vi "configure.vi"(7 "httpRequestID":u32) -> ()   [LabVIEW 2011]
doc: "This VI is a state machine that can be ran from a Browser."
uses:
  server/database/Users/User Record.ctl
  <vilib>/wsapi/NI_WebServices.lvlib
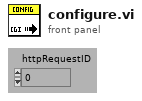
[diagram p1: front panel]
types:
  T1 = typedef "User Record.ctl" = cluster{"ixUser":i32, "sxUsername":string, "sLastName":string, "sFirstName":string, "sEmail":string, "sPassword":string, "tLoginTime":timestamp, "sLoginComputer":string, "fAdministrator":bool, "fRunSequences":bool, "fModifySequences":bool, "fRunScenarios":bool, "fModifyScenarios":bool, "fModifyTemplates":bool, "fModifyUsers":bool, "fModifyStations":bool, "fModifyFields":bool}
  T2 = typedef "Connection Refnum.ctl" = cluster{"Environment Handle":i32, "Connection Handle":i32}
  T3 = typedef "Keyed Array.ctl" = cluster{"keys":string[], "values":string[]}
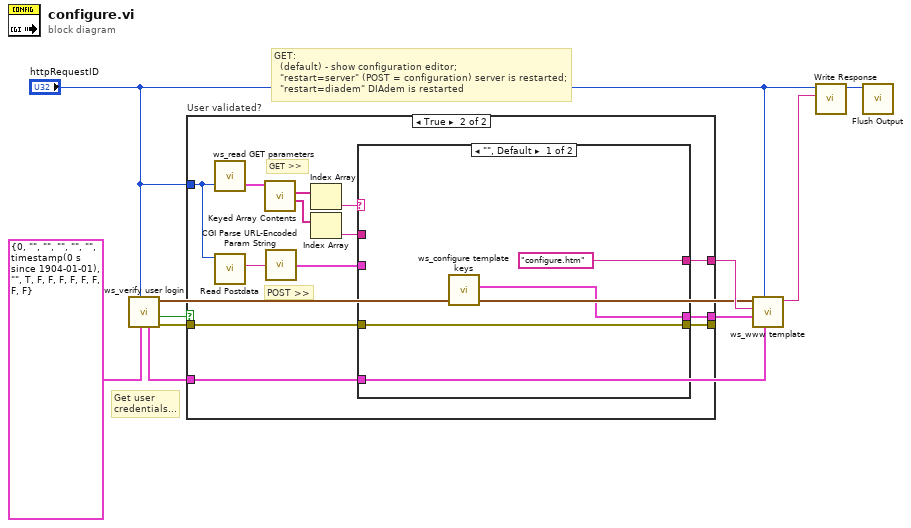
[diagram p0: block diagram]
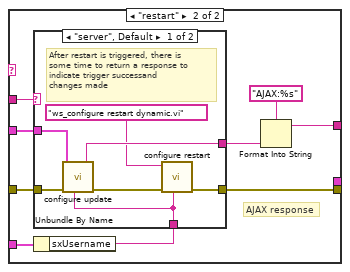
[diagram p3: hidden frame]
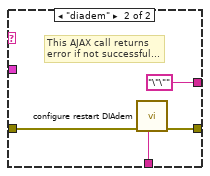
[diagram p4: hidden frame]
diagram:
  # "GET:\n  (default) - show configuration editor;\n  \"restart=server\" (POST = configuration) server is restarted;\n  \"restart=diadem\" DIAdem is restarted"
  # "Get user \ncredentials..."
  n1 = call "ws_verify user login.vi"("Required Permisions"=T1 {"ixUser"=0, "sxUsername"="", "sLastName"="", "sFirstName"="", "sEmail"="", "sPassword"="", "tLoginTime"=timestamp(0 s since 1904-01-01), "sLoginComputer"="", "fAdministrator"=TRUE, "fRunSequences"=FALSE, "fModifySequences"=FALSE, "fRunScenarios"=FALSE, "fModifyScenarios"=FALSE, "fModifyTemplates"=FALSE, "fModifyUsers"=FALSE, "fModifyStations"=FALSE, "fModifyFields"=FALSE} ("User Record"), "httpRequestID"="httpRequestID") -> ("error out"=w10:errorcluster, "User Verified\nand Spartan\nAuthorized?"=w4:bool, "DB Connection Ref"=w5:T2, "User"=w7:T1)  [unwired: 6 in]
  n2 = case "User validated?" shown="True" w4 {
    tunnel: w10 -> [w11 w16]
    tunnel: [w11 w19] -> _
    tunnel: w7 -> [_ w17]
    tunnel: [_ w15] -> w8
    tunnel: [_ w14] -> w6
    tunnel: "httpRequestID" -> [_ w13]
    frame False {
    }
    frame True {
      # "POST >>"
      # "GET >>"
      n3 = call "ws_read GET parameters.vi"("httpRequestID"=w13) -> ("GET query params"=w18:T3)  [unwired: 2 in]
      n4 = call <vilib>:"Read Postdata.vi"("httpRequestID"=w13) -> ("postdata"=w12:string)  [unwired: 8 in, 2 out]
      n5 = call <vilib>:"Keyed Array Contents.vi"("array in"=w18) -> ("values"=w21:string[], "keys"=w23:string[])  [unwired: 4 in, 1 out]
      n6 = call <vilib>:"CGI Parse URL-Encoded Param String.vi"("url-encoded param string"=w12) -> ("params"=w24:T3)
      n7 = Index Array(array=w23) -> (element=w22:string)  [unwired: 1 in]
      n8 = Index Array(array=w21) -> (element=w20:string)  [unwired: 1 in]
      n9 = case shown="\"\", Default" w22 {
        tunnel: w24 -> [_ w31]
        tunnel: w16 -> [w27 w36]
        tunnel: [w27 w35] -> w19
        tunnel: w17 -> [_ w34]
        tunnel: w20 -> [_ w32]
        tunnel: [w26 _] -> w15
        tunnel: ["configure.htm" ("Template (\"\")") w28] -> w14
        frame "", Default {
          n10 = call "ws_configure template keys.vi"() -> ("Template Keys"=w26:T3)  [unwired: 7 in]
        }
        frame "restart" {
          # "AJAX response"
          n11 = Unbundle By Name(w34) -> ("sxUsername"=w33:string)
          n12 = case shown="\"server\", Default" w32 {
            tunnel: w36 -> [w40 w47]
            tunnel: [w43 w45] -> w35
            tunnel: w33 -> [w41 w46]
            tunnel: w31 -> [w42 _]
            tunnel: [w38 "\"\"" ("Template (\"\")")] -> w30
            frame "server", Default {
              # "After restart is triggered, there is \nsome time to return a response to \nindicate trigger successand\nchanges made"
              n13 = call "configure update.vi"("Username (\"\")"=w41, "error in (no error)"=w40, "POST (empty)"=w42) -> ("error out"=w39:errorcluster, "Updates"=w38:string)  [unwired: 4 out]
              n14 = call "configure restart.vi"("UserName"=w41, "error in (no error)"=w39, "Dynamic Restart VI (\"\")"="ws_configure restart dynamic.vi") -> ("error out"=w43:errorcluster)  [unwired: 1 in, 4 out]
            }
            frame "diadem" {
              # "This AJAX call returns \nerror if not successful..."
              n15 = call "configure restart DIAdem.vi"("Username (\"\")"=w46, "error in (no error)"=w47) -> ("error out"=w45:errorcluster)  [unwired: 9 out]
            }
          }
          n16 = Format Into String(format string="AJAX:%s" ("Template (\"\")"), w30) -> (resulting string=w28:string)  [unwired: 2 in, 1 out]
        }
      }
    }
  }
  n17 = call "ws_www template.vi"("User"=w7, "httpRequestID"="httpRequestID", "Template Keys (empty)"=w8, "Template (\"\")"=w6, "DB Connection Ref"=w5) -> ("HTTP Template Content"=w2:string)  [unwired: 6 in]
  n18 = call <vilib>:"Write Response.vi"("response string"=w2, "httpRequestID"="httpRequestID") -> ("httpRequestID out"=w3:u32)  [unwired: 8 in, 1 out]
  n19 = call <vilib>:"Flush Output.vi"("httpRequestID"=w3) -> ()  [unwired: 9 in, 2 out]
